vi "Out_S6F20.vi"(8 "error in (no error)":errorcluster, 10 "Value":cluster{"Format Code":T1, "Value":variant}[](array[cluster]), 11 "S6 Message Class in":refnum<class "S6 Message Class.lvclass">) -> (0 "error out":errorcluster, 3 "S6 Message Class out":refnum<class "S6 Message Class.lvclass">)   [LabVIEW 2020, in "SECS Communication.lvlib" / "S6 Message Class.lvclass"]
uses:
  S6 Message Class.lvclass
  D:/Dropbox/SECS/SECS_GEM v1.0.6/Com/SECS Communication/SECS-II Class/SECS-II Class.lvclass
  SECS-II Class/Format Code.ctl
  SECS-II Class/Data Message_List.vi
  SECS-II Class/Variant To Data_ASCII.vi
  SECS-II Class/Data Message_ASCII.vi
  SECS-II Class/Variant To Data_Binary.vi
  SECS-II Class/Data Message_Binary.vi
  SECS-II Class/Variant To Data_Boolean.vi
  SECS-II Class/Data Message_Boolean.vi
  SECS-II Class/Variant To Data_J.vi
  SECS-II Class/Data Message_J.vi
  SECS-II Class/Variant To Data_I1.vi
  SECS-II Class/Data Message_I1 .vi
  SECS-II Class/Variant To Data_I2.vi
  SECS-II Class/Data Message_I2.vi
  SECS-II Class/Variant To Data_I4.vi
  SECS-II Class/Data Message_I4.vi
  SECS-II Class/Variant To Data_I8.vi
  SECS-II Class/Data Message_I8.vi
  SECS-II Class/Variant To Data_U1.vi
  SECS-II Class/Data Message_U1.vi
  SECS-II Class/Variant To Data_U2.vi
  SECS-II Class/Data Message_U2.vi
  SECS-II Class/Variant To Data_U4.vi
  SECS-II Class/Data Message_U4.vi
  SECS-II Class/Variant To Data_U8.vi
  SECS-II Class/Data Message_U8.vi
  SECS-II Class/Variant To Data_F4.vi
  SECS-II Class/Data Message_F4.vi
  SECS-II Class/Variant To Data_F8.vi
  SECS-II Class/Data Message_F8.vi
  SECS-II Class/Variant To Data_Character.vi
  SECS-II Class/Data Message_Character.vi
  SECS-II Class/SECS-II Class.lvclass
  D:/Dropbox/SECS/SECS_GEM v1.0.6/Com/SECS Communication/S6 Message Class/S6 Message Class.lvclass
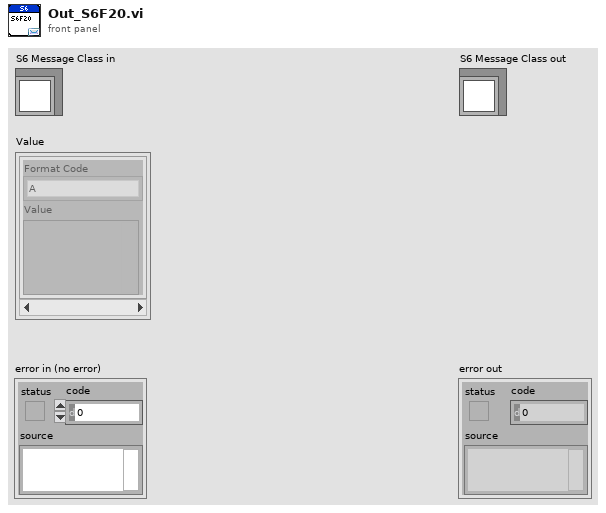
[diagram p1: front panel]
types:
  T1 = typedef "SECS Communication.lvlib/SECS-II Class.lvclass/Format Code.ctl" = enum16{"L", "A", "B", "Boolean", "J", "I1", "I2", "I4", "I8", "U1", "U2", "U4", "U8", "F4", "F8", "Char"}
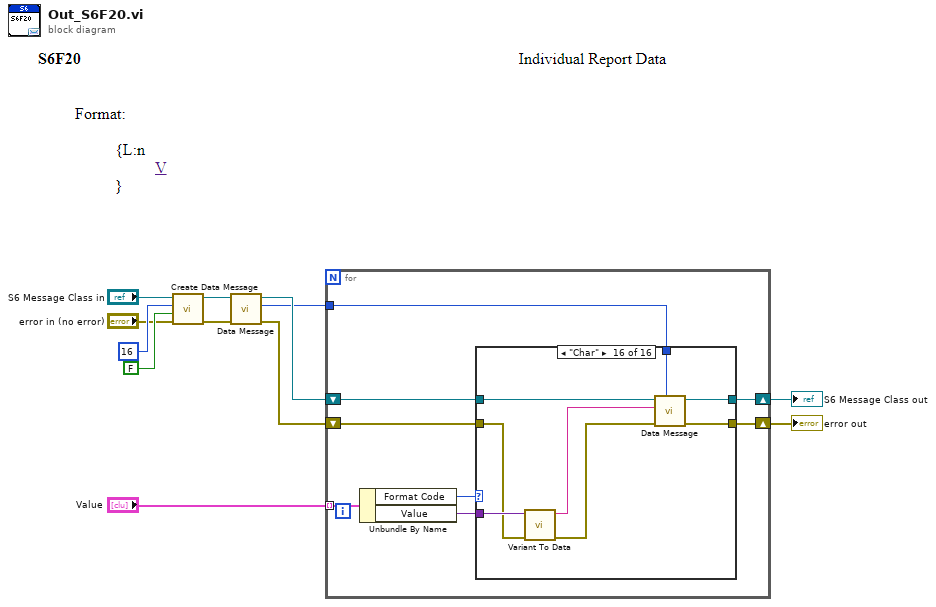
[diagram p0: block diagram]
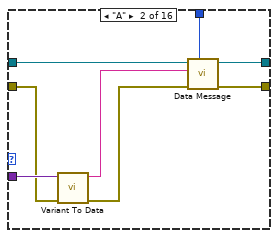
[diagram p3: hidden frame]
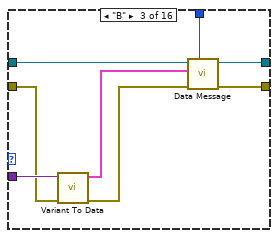
[diagram p4: hidden frame]
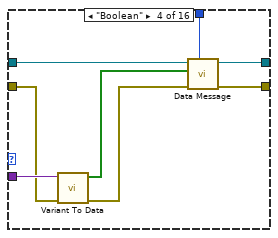
[diagram p5: hidden frame]
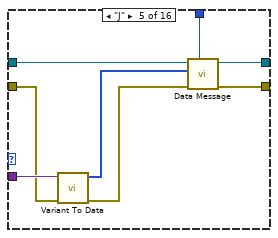
[diagram p6: hidden frame]
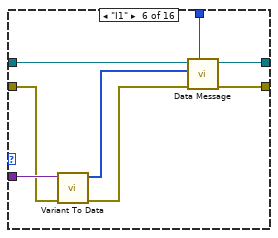
[diagram p7: hidden frame]
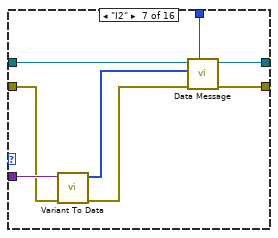
[diagram p8: hidden frame]
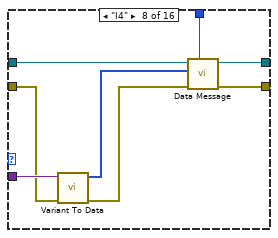
[diagram p9: hidden frame]
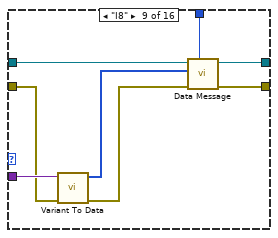
[diagram p10: hidden frame]
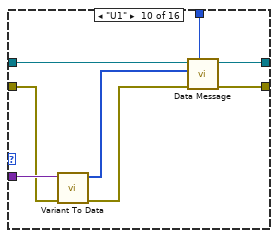
[diagram p11: hidden frame]
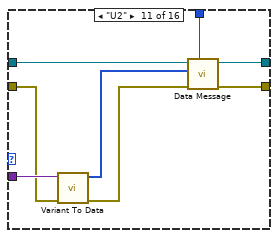
[diagram p12: hidden frame]
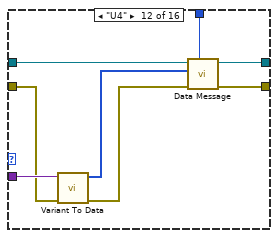
[diagram p13: hidden frame]
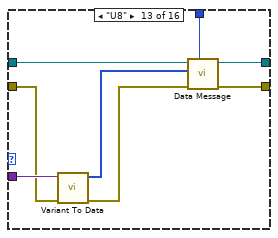
[diagram p14: hidden frame]
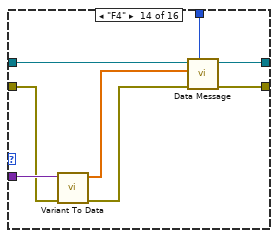
[diagram p15: hidden frame]
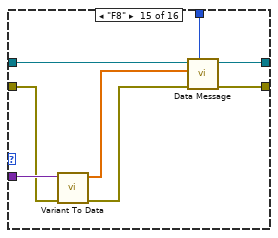
[diagram p16: hidden frame]
diagram:
  n1 = call "Create Data Message.vi"("error in (no error)"="error in (no error)", "W-Bit"=FALSE, "Function"=u8 16, "SECS-II Class in"="S6 Message Class in") -> ("error out"=w8:errorcluster, "SECS-II Class out"=w7:refnum<class "S6 Message Class.lvclass">)  [unwired: 6 in]
  n2 = call-poly "Data Message.vi"("error in"=w8, "SECS-II Class in"=w7) -> ("error out"=w4:errorcluster, "Index"=w5:i32, "SECS-II Class out"=w6:refnum<class "S6 Message Class.lvclass">)  [unwired: 7 in]
  n3 = for {
    shift-right: [w15] -> w3
    shift-left: w6 -> [w18]
    shift-right: [w14] -> w2
    shift-left: w4 -> [w19]
    tunnel: "Value" -> [w20] mode=indexing
    tunnel: w5 -> [w13]
    n4 = Unbundle By Name(w20) -> ("Format Code"=w17:T1, "Value"=w16:variant)
    n5 = case shown="\"Char\"" w17 {
      tunnel: w16 -> [_ w26 w34 w42 w50 w58 w66 w74 w82 w90 w98 w106 w114 w122 w130 w138]
      tunnel: w18 -> [w22 w30 w38 w46 w54 w62 w70 w78 w86 w94 w102 w110 w118 w126 w134 w142]
      tunnel: w19 -> [w21 w25 w33 w41 w49 w57 w65 w73 w81 w89 w97 w105 w113 w121 w129 w137]
      tunnel: [w22 w28 w36 w44 w52 w60 w68 w76 w84 w92 w100 w108 w116 w124 w132 w140] -> w15
      tunnel: [w21 w27 w35 w43 w51 w59 w67 w75 w83 w91 w99 w107 w115 w123 w131 w139] -> w14
      tunnel: w13 -> [_ w29 w37 w45 w53 w61 w69 w77 w85 w93 w101 w109 w117 w125 w133 w141]
      frame "L", Default {
      }
      frame "A" {
        n6 = call-poly "Variant To Data.vi"("error in (no error)"=w25, "Variant"=w26) -> ("error out"=w24:errorcluster, "Data"=w23:string)  [unwired: 7 in, 1 out]
        n7 = call-poly "Data Message.vi"("Parent Index"=w29, "error in"=w24, "Data"=w23, "SECS-II Class in"=w30) -> ("error out"=w27:errorcluster, "SECS-II Class out"=w28:refnum<class "S6 Message Class.lvclass">)  [unwired: 6 in]
      }
      frame "B" {
        n8 = call-poly "Variant To Data.vi"("error in (no error)"=w33, "Variant"=w34) -> ("error out"=w32:errorcluster, "Data Cluster"=w31:cluster{"Data":bool[]}[])  [unwired: 7 in, 1 out]
        n9 = call-poly "Data Message.vi"("Parent Index"=w37, "error in"=w32, "Data Cluster"=w31, "SECS-II Class in"=w38) -> ("error out"=w35:errorcluster, "SECS-II Class out"=w36:refnum<class "S6 Message Class.lvclass">)  [unwired: 6 in]
      }
      frame "Boolean" {
        n10 = call-poly "Variant To Data.vi"("error in (no error)"=w41, "Variant"=w42) -> ("error out"=w40:errorcluster, "Data"=w39:bool[])  [unwired: 7 in, 1 out]
        n11 = call-poly "Data Message.vi"("Parent Index"=w45, "error in"=w40, "Data"=w39, "SECS-II Class in"=w46) -> ("error out"=w43:errorcluster, "SECS-II Class out"=w44:refnum<class "S6 Message Class.lvclass">)  [unwired: 6 in]
      }
      frame "J" {
        n12 = call-poly "Variant To Data.vi"("error in (no error)"=w49, "Variant"=w50) -> ("error out"=w48:errorcluster, "Data"=w47:i64[])  [unwired: 7 in, 1 out]
        n13 = call-poly "Data Message.vi"("Parent Index"=w53, "error in"=w48, "Data"=w47, "SECS-II Class in"=w54) -> ("error out"=w51:errorcluster, "SECS-II Class out"=w52:refnum<class "S6 Message Class.lvclass">)  [unwired: 6 in]
      }
      frame "I1" {
        n14 = call-poly "Variant To Data.vi"("error in (no error)"=w57, "Variant"=w58) -> ("error out"=w56:errorcluster, "Data"=w55:i8[])  [unwired: 7 in, 1 out]
        n15 = call-poly "Data Message.vi"("Parent Index"=w61, "error in"=w56, "Data"=w55, "SECS-II Class in"=w62) -> ("error out"=w59:errorcluster, "SECS-II Class out"=w60:refnum<class "S6 Message Class.lvclass">)  [unwired: 6 in]
      }
      frame "I2" {
        n16 = call-poly "Variant To Data.vi"("error in (no error)"=w65, "Variant"=w66) -> ("error out"=w64:errorcluster, "Data"=w63:i16[])  [unwired: 7 in, 1 out]
        n17 = call-poly "Data Message.vi"("Parent Index"=w69, "error in"=w64, "Data"=w63, "SECS-II Class in"=w70) -> ("error out"=w67:errorcluster, "SECS-II Class out"=w68:refnum<class "S6 Message Class.lvclass">)  [unwired: 6 in]
      }
      frame "I4" {
        n18 = call-poly "Variant To Data.vi"("error in (no error)"=w73, "Variant"=w74) -> ("error out"=w72:errorcluster, "Data"=w71:i32[])  [unwired: 7 in, 1 out]
        n19 = call-poly "Data Message.vi"("Parent Index"=w77, "error in"=w72, "Data"=w71, "SECS-II Class in"=w78) -> ("error out"=w75:errorcluster, "SECS-II Class out"=w76:refnum<class "S6 Message Class.lvclass">)  [unwired: 6 in]
      }
      frame "I8" {
        n20 = call-poly "Variant To Data.vi"("error in (no error)"=w81, "Variant"=w82) -> ("error out"=w80:errorcluster, "Data"=w79:i64[])  [unwired: 7 in, 1 out]
        n21 = call-poly "Data Message.vi"("Parent Index"=w85, "error in"=w80, "Data"=w79, "SECS-II Class in"=w86) -> ("error out"=w83:errorcluster, "SECS-II Class out"=w84:refnum<class "S6 Message Class.lvclass">)  [unwired: 6 in]
      }
      frame "U1" {
        n22 = call-poly "Variant To Data.vi"("error in (no error)"=w89, "Variant"=w90) -> ("error out"=w88:errorcluster, "Data"=w87:u8[])  [unwired: 7 in, 1 out]
        n23 = call-poly "Data Message.vi"("Parent Index"=w93, "error in"=w88, "Data"=w87, "SECS-II Class in"=w94) -> ("error out"=w91:errorcluster, "SECS-II Class out"=w92:refnum<class "S6 Message Class.lvclass">)  [unwired: 6 in]
      }
      frame "U2" {
        n24 = call-poly "Variant To Data.vi"("error in (no error)"=w97, "Variant"=w98) -> ("error out"=w96:errorcluster, "Data"=w95:u16[])  [unwired: 7 in, 1 out]
        n25 = call-poly "Data Message.vi"("Parent Index"=w101, "error in"=w96, "Data"=w95, "SECS-II Class in"=w102) -> ("error out"=w99:errorcluster, "SECS-II Class out"=w100:refnum<class "S6 Message Class.lvclass">)  [unwired: 6 in]
      }
      frame "U4" {
        n26 = call-poly "Variant To Data.vi"("error in (no error)"=w105, "Variant"=w106) -> ("error out"=w104:errorcluster, "Data"=w103:u32[])  [unwired: 7 in, 1 out]
        n27 = call-poly "Data Message.vi"("Parent Index"=w109, "error in"=w104, "Data"=w103, "SECS-II Class in"=w110) -> ("error out"=w107:errorcluster, "SECS-II Class out"=w108:refnum<class "S6 Message Class.lvclass">)  [unwired: 6 in]
      }
      frame "U8" {
        n28 = call-poly "Variant To Data.vi"("error in (no error)"=w113, "Variant"=w114) -> ("error out"=w112:errorcluster, "Data"=w111:u64[])  [unwired: 7 in, 1 out]
        n29 = call-poly "Data Message.vi"("Parent Index"=w117, "error in"=w112, "Data"=w111, "SECS-II Class in"=w118) -> ("error out"=w115:errorcluster, "SECS-II Class out"=w116:refnum<class "S6 Message Class.lvclass">)  [unwired: 6 in]
      }
      frame "F4" {
        n30 = call-poly "Variant To Data.vi"("error in (no error)"=w121, "Variant"=w122) -> ("error out"=w120:errorcluster, "Data"=w119:sgl[])  [unwired: 7 in, 1 out]
        n31 = call-poly "Data Message.vi"("Parent Index"=w125, "error in"=w120, "Data"=w119, "SECS-II Class in"=w126) -> ("error out"=w123:errorcluster, "SECS-II Class out"=w124:refnum<class "S6 Message Class.lvclass">)  [unwired: 6 in]
      }
      frame "F8" {
        n32 = call-poly "Variant To Data.vi"("error in (no error)"=w129, "Variant"=w130) -> ("error out"=w128:errorcluster, "Data"=w127:dbl[])  [unwired: 7 in, 1 out]
        n33 = call-poly "Data Message.vi"("Parent Index"=w133, "error in"=w128, "Data"=w127, "SECS-II Class in"=w134) -> ("error out"=w131:errorcluster, "SECS-II Class out"=w132:refnum<class "S6 Message Class.lvclass">)  [unwired: 6 in]
      }
      frame "Char" {
        n34 = call-poly "Variant To Data.vi"("error in (no error)"=w137, "Variant"=w138) -> ("error out"=w136:errorcluster, "Data"=w135:string)  [unwired: 7 in, 1 out]
        n35 = call-poly "Data Message.vi"("Parent Index"=w141, "error in"=w136, "Data"=w135, "SECS-II Class in"=w142) -> ("error out"=w139:errorcluster, "SECS-II Class out"=w140:refnum<class "S6 Message Class.lvclass">)  [unwired: 6 in]
      }
    }
  }
  "error out" <- w2
  "S6 Message Class out" <- w3
